vi "Day 4 Debugging.vi"() -> ()   [LabVIEW 2026]
panel:
  out "Boolean":bool
  out "Area Of Triangle":dbl
  in  "Side C (cm)":dbl
  in  "Side B(cm)":dbl
  in  "Side A (cm)":dbl
  # "Area of Triangle"
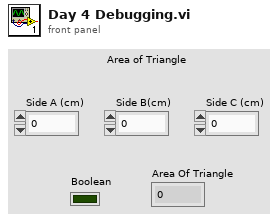
[diagram p1: front panel]
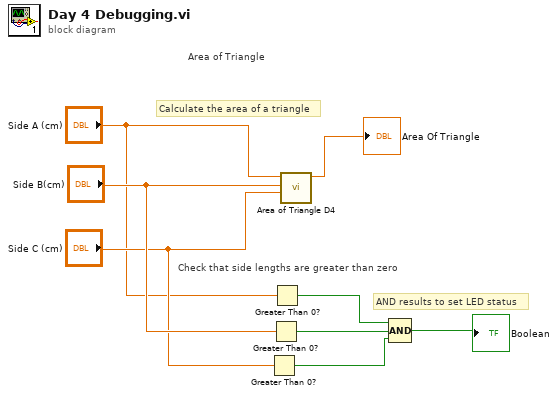
[diagram p0: block diagram]
diagram:
  # "Check that side lengths are greater than zero"
  # "Calculate the area of a triangle"
  # "AND results to set LED status"
  # "Area of Triangle"
  n1 = Greater Than 0?(x="Side C (cm)") -> (x > 0?=w2:bool)
  n2 = Greater Than 0?(x="Side B(cm)") -> (x > 0?=w5:bool)
  n3 = Greater Than 0?(x="Side A (cm)") -> (x > 0?=w6:bool)
  n4 = call "Area of Triangle D4.vi"("Side C (cm)"="Side C (cm)", "Side B(cm)"="Side B(cm)", "Side A (cm)"="Side A (cm)") -> ("Area Of Triangle"=→"Area Of Triangle":dbl)  [unwired: 8 in]
  n5 = Compound Arithmetic op=AND(w6, w5, w2) -> (→"Boolean":bool)
